vi "Read_Gripper_State.vi"(0 "error in":errorcluster, 2 "Side":T2, 3 "node":string) -> (1 "error out":errorcluster, 4 "Gripper State":T1)   [LabVIEW 2010]
doc: "Returns information from subscription to /sdk/robot/limb/<limb>/accessory/gripper/state"
uses:
  <userlib>/ROSforLV_0.1/ROS/Code/SubVIs/BaxterSide.ctl
panel:
  out "Reply":string
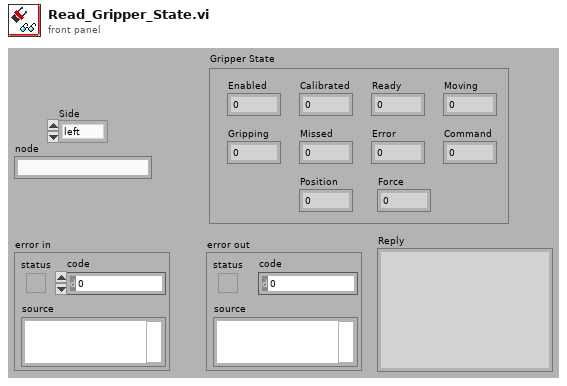
[diagram p1: front panel]
types:
  T1 = cluster{"Enabled":u8, "Calibrated":u8, "Ready":u8, "Moving":u8, "Gripping":u8, "Missed":u8, "Error":u8, "Command":u8, "Position":sgl, "Force":sgl}
  T2 = typedef "BaxterSide.ctl" = enum16{"left", "right"}
  T3 = typedef "_ROSControl.ctl" = cluster{"topic port":u16, "Node":string, "topic":string, "type":string, "node port":u32, "error ":errorcluster, "Direction":T4, "APIs":string[]}
  T4 = typedef "_ROSDirection.ctl" = enum16{"Node", "Publisher", "Subscriber", "Service Client"}
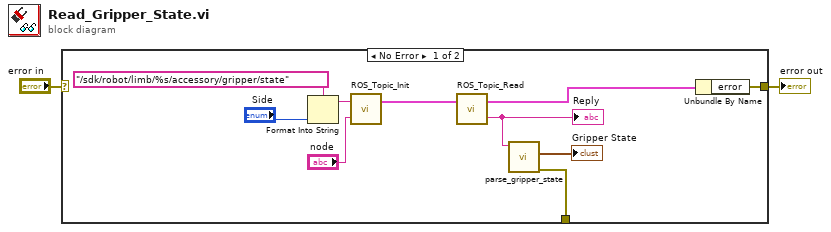
[diagram p0: block diagram]
diagram:
  n1 = case shown="No Error" "error in" {
    selector: "error in" -> [_ w13]
    tunnel: [w12 w13] -> w2
    tunnel: [w4 _] -> _
    frame No Error {
      n2 = Format Into String(format string="/sdk/robot/limb/%s/accessory/gripper/state" ("topic"), "Side") -> (resulting string=w8:string)  [unwired: 2 in, 1 out]
      n3 = call <userlib>:"ROS_Topic_Init.vi"("node"="node", "topic"=w8) -> ("ROS out"=w10:T3)  [unwired: 1 in]
      n4 = call <userlib>:"ROS_Topic_Read.vi"("ROS in"=w10) -> ("Reply"=w6:string, "ROS out"=w7:T3)  [unwired: 1 in]
      "Reply" <- w6
      n5 = call <userlib>:"parse_gripper_state.vi"("msg in"=w6) -> ("error out"=w4:errorcluster, "Gripper State"=→"Gripper State":T1)  [unwired: 4 in, 1 out]
      n6 = Unbundle By Name(w7) -> ("error"=w12:errorcluster)
    }
    frame Error {
    }
  }
  "error out" <- w2
